vi "Actor Core.vi"(8 "error in":errorcluster, 11 "Alpha UI in":refnum<class "Simulated Wash Display Console.lvclass">) -> (0 "error out":errorcluster, 3 "Actor out":refnum<class "Actor.lvclass">)   [LabVIEW 2012, in "Simulated Wash Display Console.lvlib" / "Simulated Wash Display Console.lvclass"]
doc: "(<B>Filename</B>: Actor Framework.lvlib:Actor.lvclass:Actor Core.vi)\n\nReceives messages to the actor, reacts to them, and initiates any error handling that may shut the actor down.\n\nDescendant classes may override this VI to append parallel tasks for the actor to complete while it handles messages. Overrides use the Call Parent Method node."
uses:
  Simulated Wash Display Console/Simulated Wash Display Console.lvclass
  <vilib>/ActorFramework/Actor/Actor.lvclass
  <vilib>/ActorFramework/Stop Msg/Stop Msg.lvclass
  Wash Display Console API/Wash Display Console API/Wash Display Console API.lvclass
panel:
  in  "Time Remaining":dbl format="%.2g"
  out "Vehicle Out of Position":bool
  out "Step LED Array":bool[](array[boolean])
  in  "Wash Entry":string
  # "[Covers: UI3D1]"
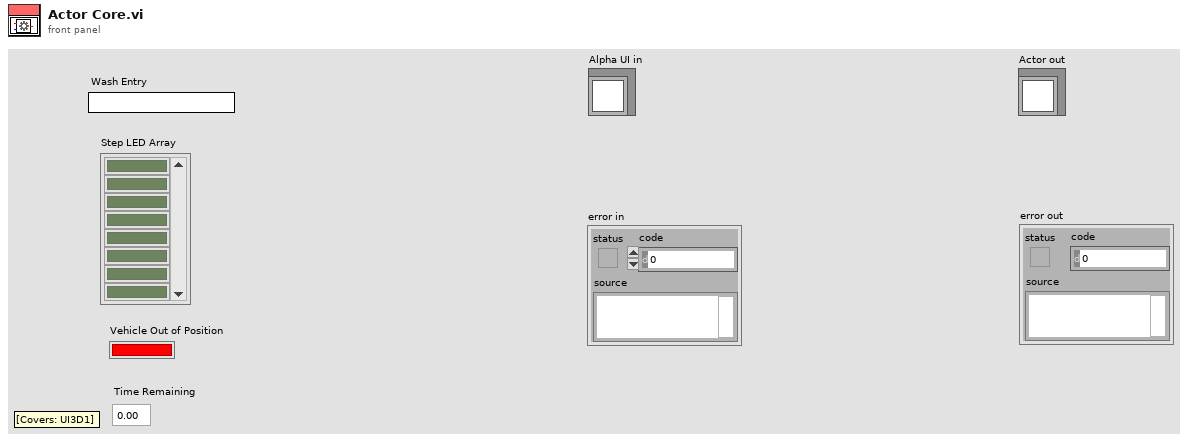
[diagram p1: front panel]
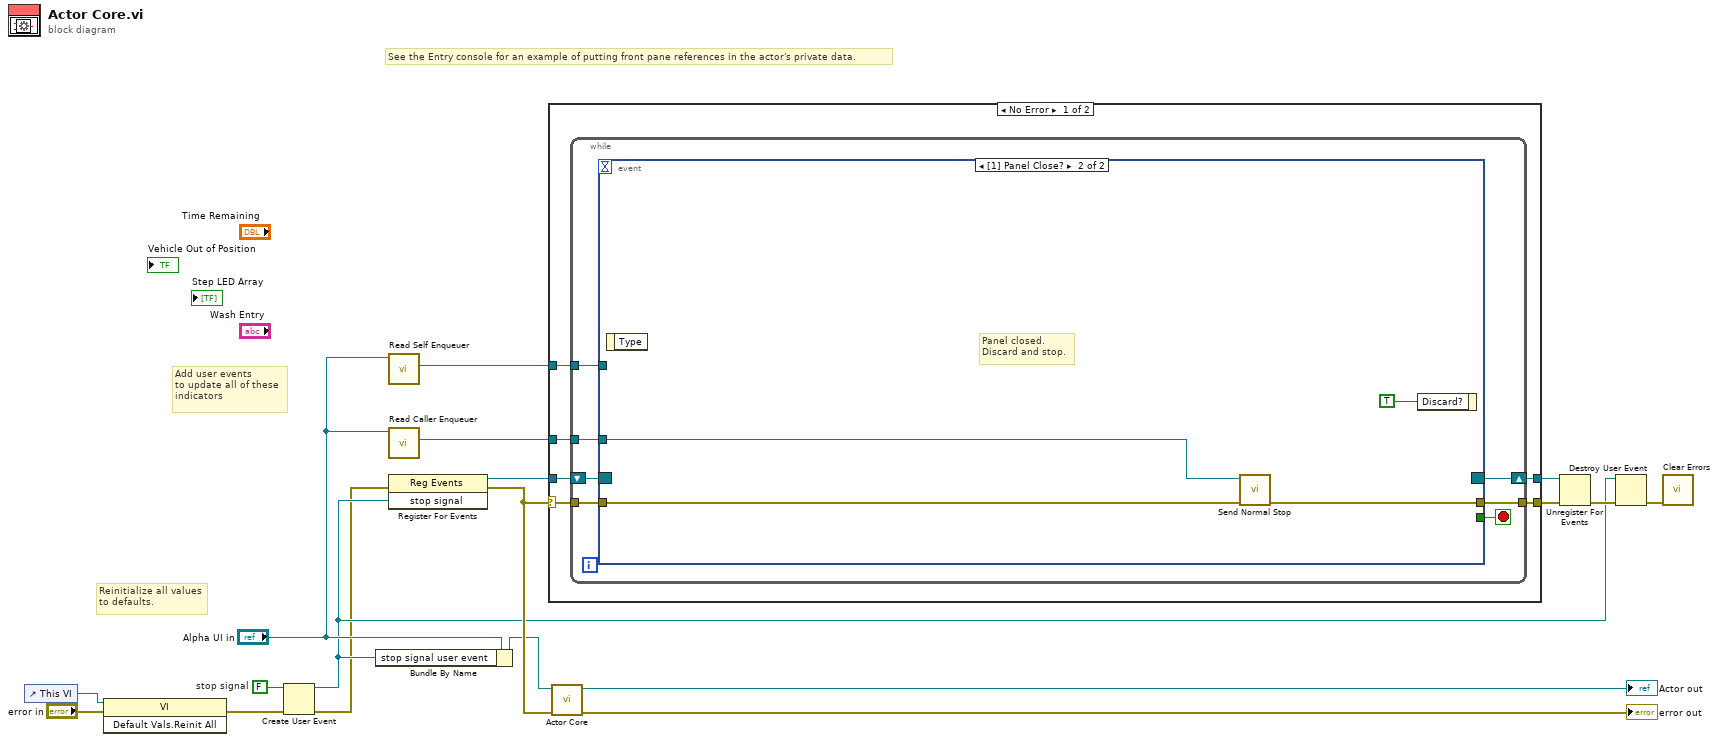
[diagram p0: block diagram]
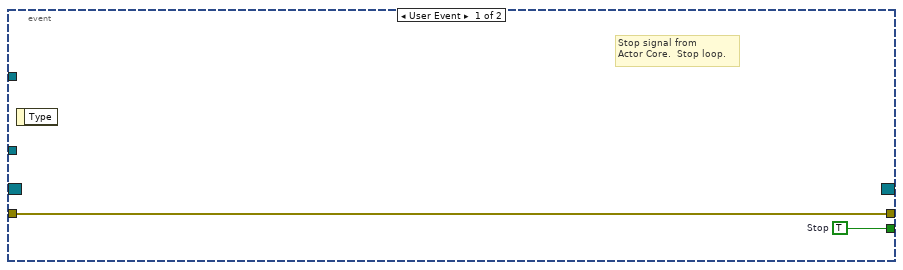
[diagram p2: hidden frame]
diagram:
  w16 = FALSE  # stop signal
  # "Add user events \nto update all of these\nindicators"
  # "See the Entry console for an example of putting front pane references in the actor's private data."
  # "Reinitialize all values\nto defaults."
  n1 = control-ref of="This VI"() -> (w6:refnum<vi>)
  n2 = invoke class="VI" method="Default Vals.Reinit All"(reference=w6, error in="error in") -> (error out=w4:errorcluster)  [unwired: 1 in, 2 out]
  n3 = Create User Event(user event datatype=w16, error in=w4) -> (user event=w7:refnum<user-event>, error out=w3:errorcluster)
  n4 = Bundle By Name(cluster="Alpha UI in", "stop signal user event"=w7) -> (w1:refnum<class "Simulated Wash Display Console.lvclass">)
  n5 = call <vilib>:"Read Self Enqueuer.vi"("Actor"="Alpha UI in") -> ("Self Enqueuer"=w18:refnum<class "Message Enqueuer.lvclass">)  [unwired: 10 in]
  n6 = call <vilib>:"Read Caller Enqueuer.vi"("Actor"="Alpha UI in") -> ("Caller Enqueuer"=w17:refnum<class "Message Enqueuer.lvclass">)  [unwired: 10 in]
  n7 = register-events(error in=w3, w7) -> (reference out=w15:refnum<event-registration>, error out=w12:errorcluster)  [unwired: 1 in]
  n8 = case shown="No Error" w12 {
    selector: w12 -> [w19 w38]
    tunnel: w18 -> [w24 _]
    tunnel: w17 -> [w23 _]
    tunnel: w15 -> [w22 w39]
    tunnel: [w21 w39] -> w13
    tunnel: [w20 w38] -> w11
    frame No Error {
      n9 = while {
        tunnel: w24 -> [w30]
        tunnel: w23 -> [w29]
        shift-right: [w27] -> w21
        shift-left: w22 -> [w28]
        tunnel: [w26] -> w20
        tunnel: w19 -> [w25]
        stop <- w31 stop-if-true
        n10 = event shown="[1] Panel Close?" {
          selector: w28 -> [_ _]
          dyn-events: [_ _] -> w27
          timeout: _ -> [_ _]
          tunnel: [w33 _] -> w31
          tunnel: w30 -> [_ _]
          tunnel: w29 -> [_ w37]
          tunnel: [w32 w36] -> w26
          tunnel: w25 -> [w32 w35]
          event User Event {
            w33 = TRUE  # Stop
            # "Stop signal from\nActor Core.  Stop loop."
            n11 = event-data() -> ()  [unwired: 1 in, 1 out]
          }
          event Panel Close? {
            # "Panel closed.\nDiscard and stop."
            n12 = event-data() -> ()  [unwired: 1 in, 1 out]
            n13 = call <vilib>:"Send Normal Stop.vi"("error in (no error)"=w35, "Message Enqueuer"=w37) -> ("error out"=w36:errorcluster)  [unwired: 9 in]
            n14 = event-data("Discard?"=TRUE) -> ()  [unwired: 1 in, 1 out]
          }
        }
      }
    }
    frame Error {
    }
  }
  n15 = call-parent "Actor Core.vi"("error in"=w12, "Actor in"=w1) -> ("error out"=→"error out":errorcluster, "Actor out"=→"Actor out":refnum<class "Actor.lvclass">)  [unwired: 8 in]
  n16 = Unregister For Events(event registration refnum=w13, error in=w11) -> (error out=w14:errorcluster)
  n17 = Destroy User Event(user event=w7, error in=w14) -> (error out=w2:errorcluster)
  n18 = call <vilib>:"Clear Errors.vi"("error in (no error)"=w2) -> ()  [unwired: 5 in, 2 out]
